vi "resultsRowAssemble.vi"(4 "Ch Values In":string[](array[string]), 5 "Ch Names In":string[](array[string]), 6 "ErrorStringIn":string, 10 "RowChValuesIn":string[](array[string]), 11 "RowChNamesIn":string[](array[string])) -> (1 "RowChValuesOut":string[](array[string]), 3 "rowChNamesOut":string[](array[string]))   [LabVIEW 2022 SP3]
uses:
  Globals/Meas_global.vi
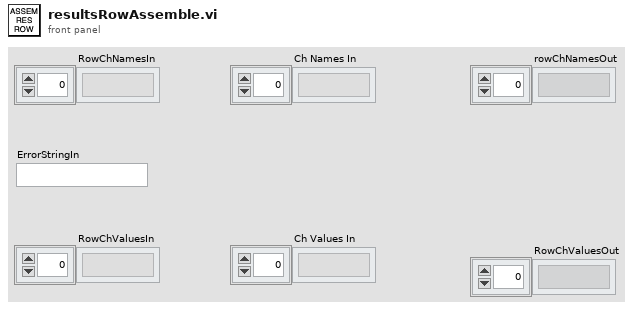
[diagram p1: front panel]
types:
  T1 = typedef "Post_Process.ctl" = enum16{"Take New Data", "Post Process Raw Data File"}
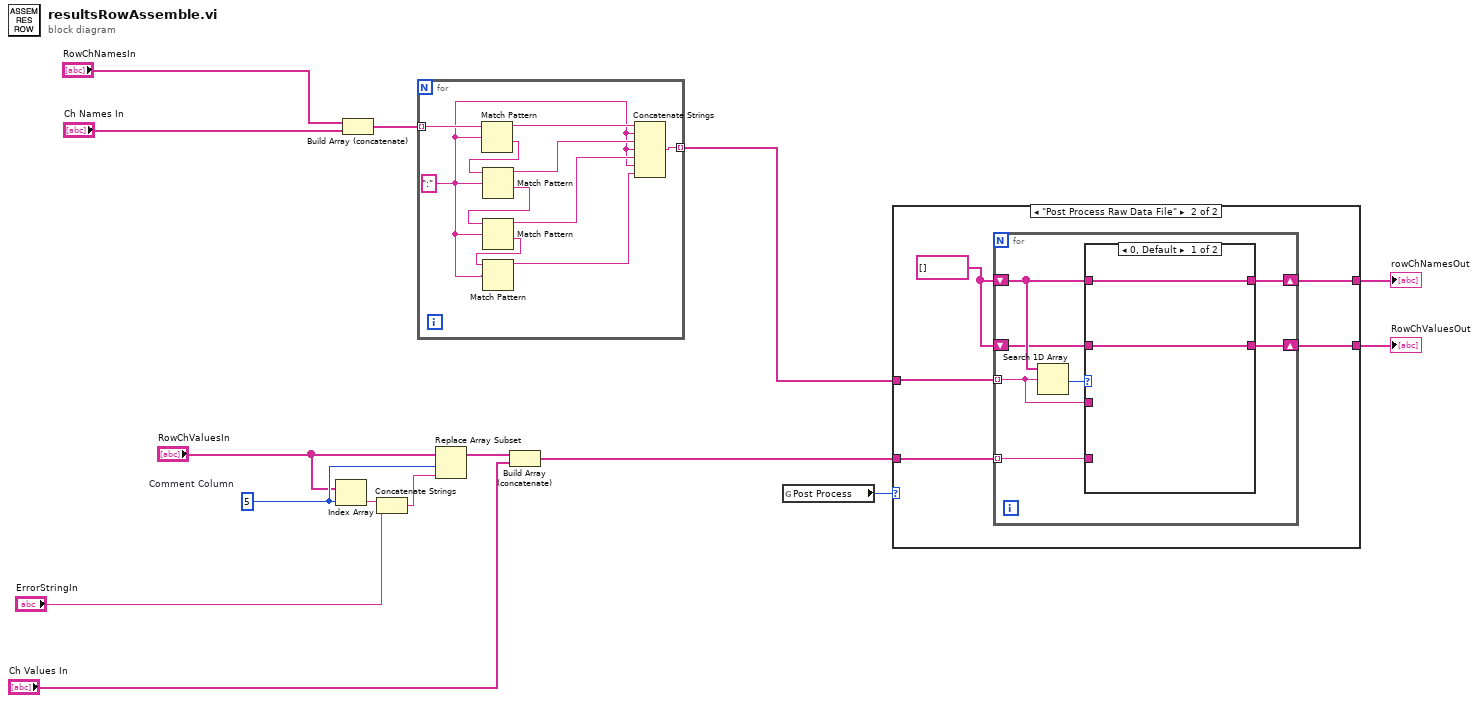
[diagram p0: block diagram]
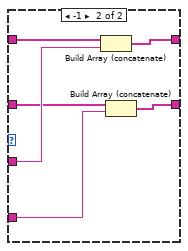
[diagram p3: hidden frame]
diagram:
  w8 = 5  # Comment Column
  n1 = Index Array(array="RowChValuesIn", index=w8) -> (element=w5:string)
  n2 = Build Array (concatenate)("RowChNamesIn", "Ch Names In") -> (w9:string[])
  n3 = Concatenate Strings(w5, "ErrorStringIn") -> (w6:string)
  n4 = for {
    tunnel: w9 -> [w19] mode=indexing
    tunnel: [w20] -> w14 mode=indexing
    w17 = ":" ("regular expression")
    n5 = Match Pattern(string=w19, regular expression=w17) -> (before substring=w23:string, after substring=w25:string)  [unwired: 3 out]
    n6 = Match Pattern(string=w25, regular expression=w17) -> (before substring=w22:string, after substring=w24:string)  [unwired: 3 out]
    n7 = Match Pattern(string=w24, regular expression=w17) -> (before substring=w21:string, after substring=w18:string)  [unwired: 3 out]
    n8 = Match Pattern(string=w18, regular expression=w17) -> (before substring=w16:string)  [unwired: 4 out]
    n9 = Concatenate Strings(w23, w17, w22, w17, w21, w17, w16) -> (w20:string)
  }
  n10 = Replace Array Subset(array="RowChValuesIn", new element=w6, index=w8) -> (w4:string[])
  n11 = Build Array (concatenate)(w4, "Ch Values In") -> (w15:string[])
  n12 = global read "Meas_global.vi" "Post Process"() -> (w11:T1)
  n13 = case shown="\"Post Process Raw Data File\"" w11 {
    tunnel: [w27 w31] -> w12
    tunnel: w14 -> [w27 w32]
    tunnel: [w26 w30] -> w13
    tunnel: w15 -> [w26 w29]
    frame "Take New Data" {
    }
    frame "Post Process Raw Data File" {
      w28 = string[] []
      n14 = for {
        shift-right: [w37] -> w31
        shift-left: w28 -> [w38]
        shift-right: [w34] -> w30
        shift-left: w28 -> [w35]
        tunnel: w32 -> [w36] mode=indexing
        tunnel: w29 -> [w33] mode=indexing
        n15 = Search 1D Array(1D array=w38, element=w36) -> (index of element=w39:i32)  [unwired: 1 out]
        n16 = case shown="0, Default" w39 {
          tunnel: w38 -> [w41 w47]
          tunnel: [w41 w46] -> w37
          tunnel: w36 -> [_ w45]
          tunnel: w35 -> [w40 w44]
          tunnel: [w40 w43] -> w34
          tunnel: w33 -> [_ w42]
          frame 0, Default {
          }
          frame -1 {
            n17 = Build Array (concatenate)(w47, w45) -> (w46:string[])
            n18 = Build Array (concatenate)(w44, w42) -> (w43:string[])
          }
        }
      }
    }
  }
  "RowChValuesOut" <- w13
  "rowChNamesOut" <- w12
